vi "Problem 20.vi"() -> ()   [LabVIEW 2013, in "Problem 20.lvlib"]
uses:
  Problem 20.lvlib
panel:
  out "Sum of Digits":i32
  out "x!":string
  in  "x!":i32
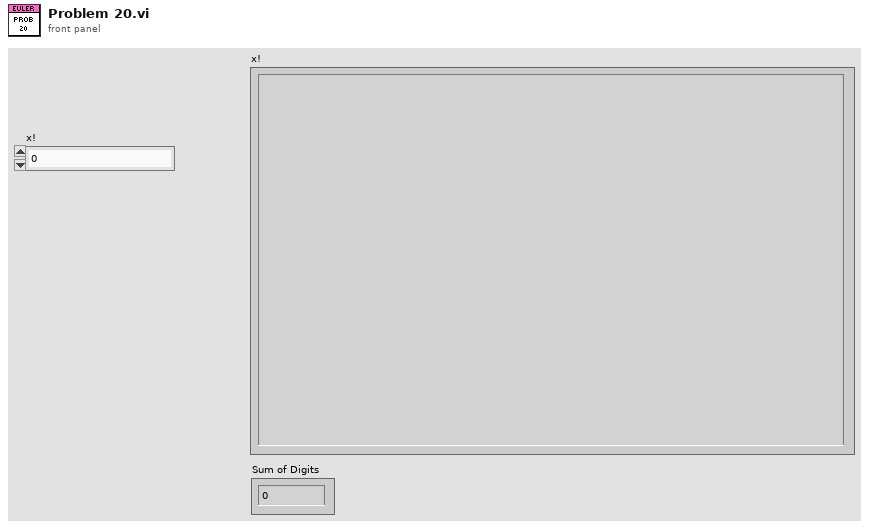
[diagram p1: front panel]
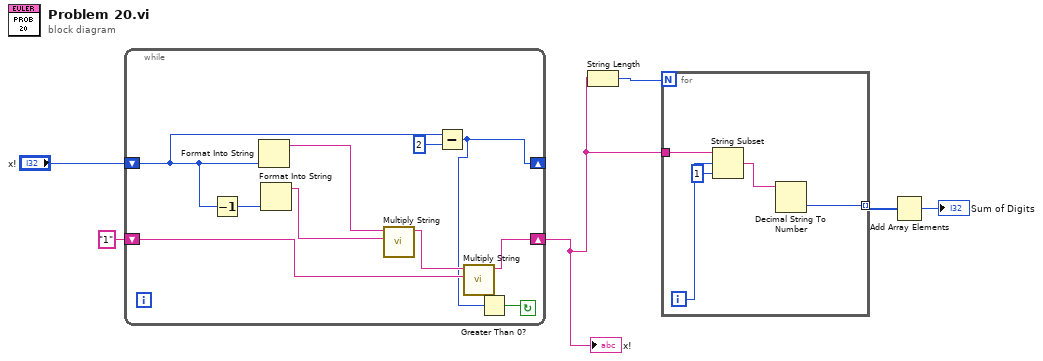
[diagram p0: block diagram]
diagram:
  n1 = while {
    shift-right: [w12] -> w3
    shift-left: "1" ("x + y") -> [w13]
    shift-right: [w7] -> _
    shift-left: "x!" -> [w10]
    stop <- w8 continue-if-true
    n2 = Decrement(x=w10) -> (x-1=w11:i32)
    n3 = Format Into String(w10) -> (resulting string=w16:string)  [unwired: 3 in, 1 out]
    n4 = Format Into String(w11) -> (resulting string=w15:string)  [unwired: 3 in, 1 out]
    n5 = call "Multiply String.vi"("y"=w15, "x"=w16) -> ("x * y"=w14:string)  [unwired: 9 in]
    n6 = Subtract(x=w10, y=2) -> (x-y=w7:i32)
    n7 = call "Multiply String.vi"("y"=w13, "x"=w14) -> ("x * y"=w12:string)  [unwired: 9 in]
    n8 = Greater Than 0?(x=w7) -> (x > 0?=w8:bool)
  }
  "x!" <- w3
  n9 = String Length(string=w3) -> (length=w4:i32)
  n10 = for {
    N: w4 -> [_]
    tunnel: w3 -> [w21]
    tunnel: [w17] -> w2 mode=indexing
    i -> [w20]
    n11 = String Subset(string=w21, offset (0)=w20, length (rest)=1 ("length (rest)")) -> (substring=w18:string)
    n12 = Decimal String To Number(string=w18) -> (number=w17:i32)  [unwired: 2 in, 1 out]
  }
  n13 = Add Array Elements(numeric array=w2) -> (sum=→"Sum of Digits":i32)
